vi "Robot Global Data.vi"() -> ()   [LabVIEW 2015]
doc: "This global VI can contain as many global variables as you need. Place a control on the panel, give it a good name. To read or write to it from a VI, drag the icon to the diagram of that VI. You can also drag from the project. Click on the node to change which global you access. You shouldn't have multiple locations writing to a global or it will cause a race-condition."
uses:
  <vilib>/Rock Robotics/WPI/Camera/WPI_CameraImageSize.ctl
  <vilib>/Rock Robotics/WPI/DriverStation/WPI_DriverStationRobotMode2.ctl
panel:
  in  "arm speed shovel":dbl=0.38
  in  "arm speed normal":dbl=0.33
  out "finishedRtweak":bool
  out "finishedLtweak":bool
  in  "Starting Position":i32=2
  in  "Defense to Cross":i32=5
  out "arm shot spot":dbl=0.39499999999999996
  out "4?":bool
  out "1-Button 8":bool
  out "1-Button 5":bool
  out "arm pot unfiltered":dbl=0.7379995469532098
  in  "cheval pos":dbl=0.475
  in  "Heading":dbl=354.51
  in  "Pitch":dbl=2.48
  in  "Yaw":dbl=-5.48
  in  "IsPracticeBot?":bool=TRUE
  in  "IR dist to CDF":dbl=0.021972654
  in  "left num":i8
  in  "climb num":i32
  in  "right num":i8
  in  "arm speed slow":dbl=0.1
  in  "arm slow spot":dbl=0.07
  in  "Left 2":bool
  in  "Right 2":bool
  in  "arm out":dbl=0.1
  in  "arm speed":dbl=0.33
  in  "IR dist threshold":dbl=2.0
  in  "IR dist to ball":dbl=0.29296872
  out "retainer override":bool
  in  "retainer num":i16=2
  in  "in ctl num":i16
  out "in pos override":bool
  in  "arm override":bool
  in  "arm start":dbl=0.745
  in  "arm extended":dbl=0.345
  in  "climb":bool
  out "PTO speed":dbl
  in  "Shoot!":bool
  in  "In ctl 2":bool=TRUE
  in  "In ctl 1":bool
  in  "In pos":bool=TRUE
  in  "Retainer 2":bool=TRUE
  in  "Retainer":bool=TRUE
  in  "Right":bool
  in  "Left":bool
  in  "climb 2":bool
  out "center Y":dbl=-0.7041666666666666
  out "center X":dbl=0.11250000000000004
  out "Distance (cam)":dbl=16.78099671253925
  in  "Shot Selector":bool
  out "arm pot":dbl=0.7372340202179969
  in  "Arm Control":dbl(knob)=1.0 scale=-1.0..1.0
  out "shift state":bool=TRUE
  in  "PTO Engaged":bool
  out "Shift Lockout?":bool
  out "Distance (enc.)":dbl=309.073629375
  out "Velocity":dbl
  out "1-Slider":dbl=0.8188976377952756
  out "1-Trigger":bool
  out "1-TopRight":bool
  out "1-TopLeft":bool
  out "1-Zrotate":dbl
  out "1-X":dbl
  out "1-Y":dbl
  out "1-TopCenter":bool
  in  "Robot Mode":T1=enum."Teleop Disabled"
  in  "image size":T2=enum."320x240"
  in  "Enable Vision":bool
  # "Arm extended = porticullus setting"
  # "Comp = 0.330\nPractice = 0.350"
  # "Tape Measures"
  # "Comp = 0.722\nPractice =  0.725"
  # "00        - normal\n01 10   - PTO engaged\n11        - climb"
  # "00        - out\n01 10   - off\n11        - in"
  # "00        - off\n01 10   - on\n11        - auto"
  # "Close"
  # "Down"
  # "Up"
  # "Far"
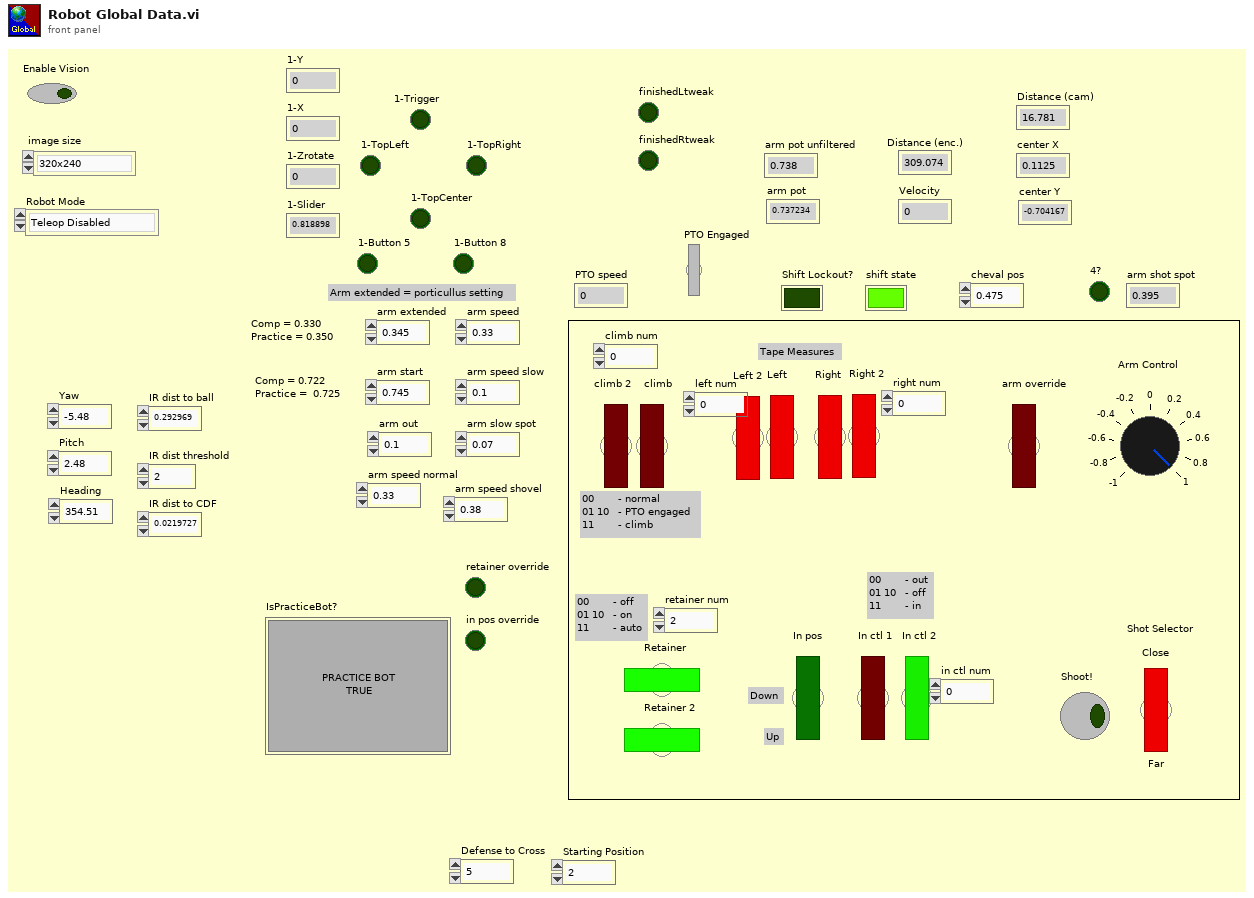
[diagram p1: front panel]
types:
  T1 = typedef "WPI_DriverStationRobotMode2.ctl" = enum16{"Autonomous Disabled", "Autonomous Enabled", "Teleop Disabled", "Teleop Enabled", "Disconnected", "Finish", "Test Disabled", "Test Enabled", "Emergency Stopped"}
  T2 = typedef "WPI_CameraImageSize.ctl" = enum16{"640x480", "320x240", "160x120", "Custom"}
diagram:
